vi "DepthSense Destroy.vi"(8 "error in (no error)":errorcluster, 11 "callbacks":cluster{"References":T1, "References":T1}) -> (0 "error out":errorcluster)   [LabVIEW 2011]
uses:
  FunctionPointerProxy/LabVIEW/t_CallbackReferences.ctl
  C:/Users/Behavior Room/Desktop/Kinect Mouse/DepthSense/FunctionPointerProxy/FunctionPointerProxy/bin/Release/FunctionPointerProxy.dll
  FunctionPointerProxy/FunctionPointerProxy/bin/Release/FunctionPointerProxy.dll
  <userlib>/libOptrima-2-3/libOptrima-2-3.lvlib
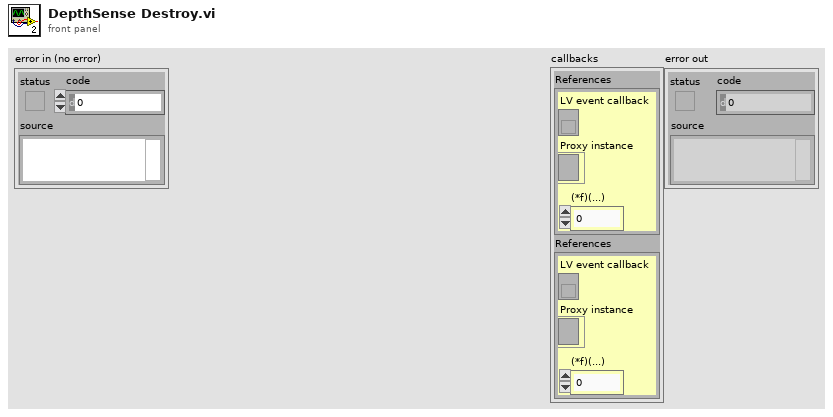
[diagram p1: front panel]
types:
  T1 = typedef "t_CallbackReferences.ctl" = cluster{"LV event callback ":refnum<k27>, "Proxy instance":refnum<k24>, "(*f)(...)":i32}
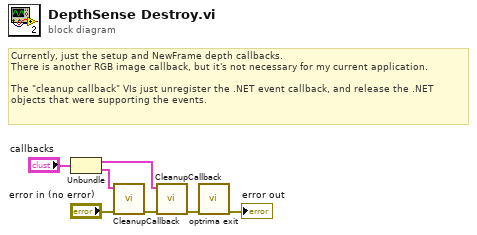
[diagram p0: block diagram]
diagram:
  # "Currently, just the setup and NewFrame depth callbacks.\nThere is another RGB image callback, but it's not necessary for my current application.\n\nThe \"cleanup callback\" VIs just unregister the .NET event callback, and release the .NET\nobjects that were supporting the events."
  n1 = Unbundle("callbacks") -> ("References"=w3:T1, "References"=w2:T1)
  n2 = call "CleanupCallback.vi"("error in (no error)"="error in (no error)", "References"=w2) -> ("error out"=w6:errorcluster)  [unwired: 9 in]
  n3 = call "CleanupCallback.vi"("error in (no error)"=w6, "References"=w3) -> ("error out"=w7:errorcluster)  [unwired: 9 in]
  n4 = call <userlib>:"optrima exit.vi"("error in (no error)"=w7) -> ("error out"=→"error out":errorcluster)  [unwired: 10 in]
